vi "HandleJoystickButtons.vi"(11 "JoystickButton":bool) -> (3 "output":bool)   [LabVIEW 2012]
uses:
  JoystickDirection.ctl
panel:
  out "Iteration":i32
  out "Current State":string
  in  "Wait (ms)":u32=11
  in  "stop":bool
  out "Direction":T1
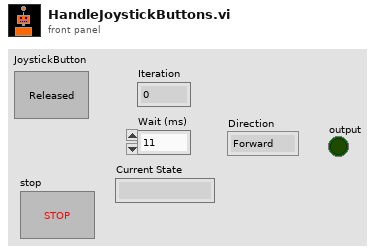
[diagram p1: front panel]
types:
  T1 = typedef "JoystickDirection.ctl" = enum16{"Forward", "Reverse"}
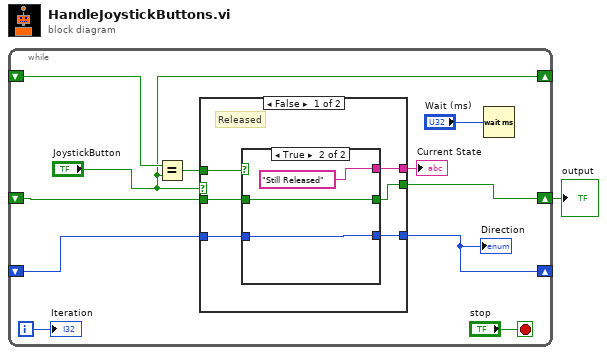
[diagram p0: block diagram]
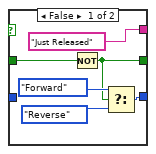
[diagram p2: hidden frame]
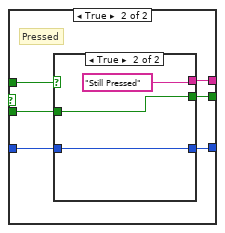
[diagram p3: hidden frame]
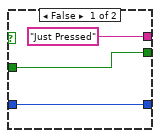
[diagram p4: hidden frame]
diagram:
  n1 = while {
    shift-right: [w8] -> w1
    shift-left: _ -> [w7]
    shift-right: ["JoystickButton"] -> _
    shift-left: _ -> [w11]
    shift-right: [w6] -> _
    shift-left: _ -> [w5]
    i -> [w2]
    stop <- "stop" stop-if-true
    n2 = Equal?(x=w11, y="JoystickButton") -> (x = y?=w9:bool)
    n3 = case shown="False" "JoystickButton" {
      tunnel: w9 -> [w18 w33]
      tunnel: [w15 w32] -> w8
      tunnel: w7 -> [w17 w31]
      tunnel: [w16 w29] -> w6
      tunnel: w5 -> [w14 w30]
      tunnel: [w13 w28] -> w3
      frame False {
        # "Released"
        n4 = case shown="True" w18 {
          tunnel: [w20 w27] -> w15
          tunnel: w17 -> [w24 w27]
          tunnel: [w21 w26] -> w16
          tunnel: w14 -> [_ w26]
          tunnel: ["Just Released" "Still Released"] -> w13
          frame False {
            n5 = Not(x=w24) -> (.not. x?=w20:bool)
            n6 = Select(t=JoystickDirection."Forward" ("Direction"), s=w20, f=JoystickDirection."Reverse" ("Direction")) -> (s? t:f=w21:T1)
          }
          frame True {
          }
        }
      }
      frame True {
        # "Pressed"
        n7 = case shown="True" w33 {
          tunnel: [w36 w39] -> w32
          tunnel: w31 -> [w36 w39]
          tunnel: [w35 w38] -> w29
          tunnel: w30 -> [w35 w38]
          tunnel: ["Just Pressed" "Still Pressed"] -> w28
          frame False {
          }
          frame True {
          }
        }
      }
    }
    "Direction" <- w6
    "Current State" <- w3
    n8 = Wait (ms)(milliseconds to wait="Wait (ms)") -> ()  [unwired: 1 out]
    "Iteration" <- w2
  }
  "output" <- w1
